vi "NI OCR-Start Training.vi"(8 "error in":errorcluster, 11 "Buffer Data In":T1={"VI Refnum"=refnum, "Src Image"=refnum, "Dst Image"=refnum, "Ctl Refnum []"=[], "Ctl Label"=[], "User Event"=refnum, "Event Registration Refnum"=refnum, "Timeout"=0, "IMAQ OCR Session"=refnum, "Objects"=[], "ROI Descriptor"={"Global Rectangle"=[], "Contours"=[]}, "Settings"={"Objects"=0, "Threshold"=128, "Reject Border"=FALSE, "Fill Holes"=FALSE, "Min Object Size"=FALSE, "Min Size"=3, "Max Object Size"=FALSE, "Max Size"=100, "Show Search Area"=FALSE, "Show Center"=TRUE, "Show Bounding Box"=TRUE}} {"Settings"."Objects" items=["Bright Objects", "Dark Objects"]; "Settings"."Threshold" min=1 max=999999999 step=1; "Settings"."Max Size" min=1 max=999999999 step=1; "Settings"."Min Size" min=1 max=999999999 step=1; "ROI Descriptor"."Contours"."Type" items=["No Selection", "Point", "Line", "Rectangle", "Oval", "Polygon", "Freehand Region", "Annulus", "Unused2", "Unused3", "Broken Line", "Freehand Line", "Rotated Rectangle"]; "Objects"."Aspect Ratio" format="%.2f"; "Objects"."Orientation" format="%.2f"; "Objects"."Area" format="%.2f"; "Objects"."Object Center"."Y" format="%.2f"; "Objects"."Object Center"."X" format="%.2f"}) -> (0 "error out":errorcluster, 3 "Buffer Data Out":T1={"VI Refnum"=refnum, "Src Image"=refnum, "Dst Image"=refnum, "Ctl Refnum []"=[], "Ctl Label"=[], "User Event"=refnum, "Event Registration Refnum"=refnum, "Timeout"=0, "IMAQ OCR Session"=refnum, "Objects"=[], "ROI Descriptor"={"Global Rectangle"=[], "Contours"=[]}, "Settings"={"Objects"=0, "Threshold"=128, "Reject Border"=FALSE, "Fill Holes"=FALSE, "Min Object Size"=FALSE, "Min Size"=3, "Max Object Size"=FALSE, "Max Size"=100, "Show Search Area"=FALSE, "Show Center"=TRUE, "Show Bounding Box"=TRUE}} {"Settings"."Objects" items=["Bright Objects", "Dark Objects"]; "Settings"."Threshold" min=1 max=999999999 step=1; "Settings"."Max Size" min=1 max=999999999 step=1; "Settings"."Min Size" min=1 max=999999999 step=1; "ROI Descriptor"."Contours"."Type" items=["No Selection", "Point", "Line", "Rectangle", "Oval", "Polygon", "Freehand Region", "Annulus", "Unused2", "Unused3", "Broken Line", "Freehand Line", "Rotated Rectangle"]; "Objects"."Aspect Ratio" format="%.2f"; "Objects"."Orientation" format="%.2f"; "Objects"."Area" format="%.2f"; "Objects"."Object Center"."Y" format="%.2f"; "Objects"."Object Center"."X" format="%.2f"})   [LabVIEW 2016]
uses:
  Data Def/NI OCR-Buffer Data.ctl
  <vilib>/vision/Image Controls.llb/IMAQ Image.ctl
  Data Def/NI OCR-User Event Data.ctl
  <vilib>/vision/OCR.llb/IMAQ OCR Session.ctl
  <vilib>/vision/NI_Vision_Development_Module.lvlib
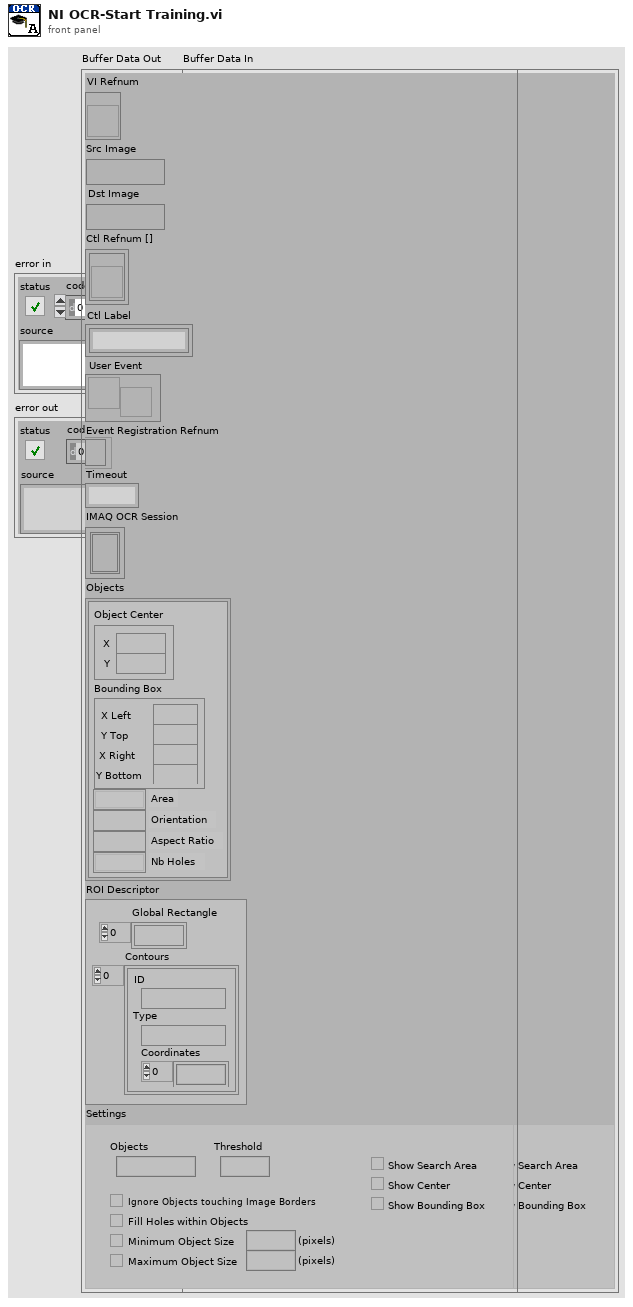
[diagram p1: front panel]
types:
  T1 = typedef "NI OCR-Buffer Data.ctl" = cluster{"VI Refnum":refnum<vi>, "Src Image":T2, "Dst Image":T2, "Ctl Refnum []":refnum<vi>[], "Ctl Label":string[], "User Event":refnum<user-event>, "Event Registration Refnum":refnum<event-registration>, "Timeout":i32, "IMAQ OCR Session":T3, "Objects":cluster{"Object Center":cluster{"X":sgl, "Y":sgl}, "Bounding Box":cluster{"X Left":i32, "Y Top":i32, "X Right":i32, "Y Bottom":i32}, "Area":sgl, "Orientation":sgl, "Aspect Ratio":sgl, "Nb Holes":i32}[], "ROI Descriptor":T4, "Settings":cluster{"Objects":u16, "Threshold":i32, "Reject Border":bool, "Fill Holes":bool, "Min Object Size":bool, "Min Size":i32, "Max Object Size":bool, "Max Size":i32, "Show Search Area":bool, "Show Center":bool, "Show Bounding Box":bool}}
  T2 = typedef "IMAQ Image.ctl" = refnum<image>
  T3 = typedef "IMAQ OCR Session.ctl" = refnum<k1>
  T4 = typedef "ROI Descriptor" = cluster{"Global Rectangle":i32[], "Contours":cluster{"ID":enum32{"External", "Internal"}, "Type":u32, "Coordinates":i32[]}[]}
  T5 = cluster{"Object Center":cluster{"X":sgl, "Y":sgl}, "Bounding Box":cluster{"X Left":i32, "Y Top":i32, "X Right":i32, "Y Bottom":i32}, "Area":sgl, "Orientation":sgl, "Aspect Ratio":sgl, "Nb Holes":i32}[]
  T6 = cluster{"X Left":i32, "Y Top":i32, "X Right":i32, "Y Bottom":i32}
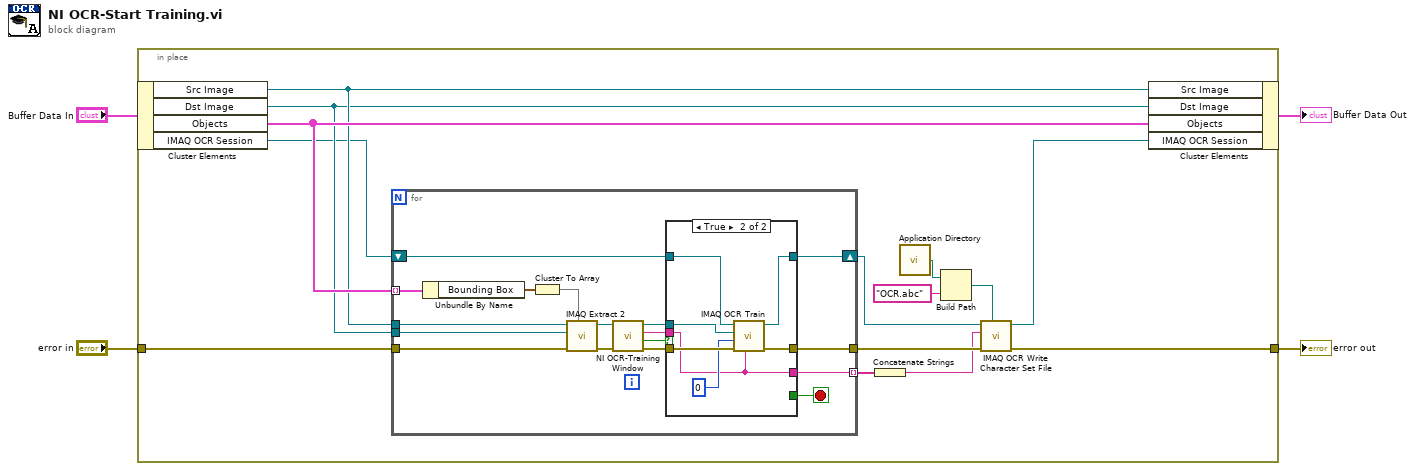
[diagram p0: block diagram]
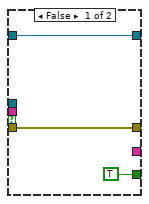
[diagram p2: hidden frame]
diagram:
  n1 = in-place {
    in-place-border: "error in" -> [w17]
    in-place-border: [w7] -> w1
    n2 = in-place-cluster #1("Buffer Data In") -> ("Src Image"=w16:T2, "Dst Image"=w15:T2, "Objects"=w18:T5, "IMAQ OCR Session"=w14:T3)
    n3 = for {
      tunnel: w18 -> [w35] mode=indexing
      tunnel: w17 -> [w34]
      tunnel: w16 -> [w32]
      tunnel: w15 -> [w33]
      shift-right: [w21] -> w10
      shift-left: w14 -> [w28]
      tunnel: [w20] -> w11
      tunnel: [w19] -> w6 mode=indexing
      stop <- w22 stop-if-true
      n4 = Unbundle By Name(w35) -> ("Bounding Box"=w31:T6)
      n5 = Cluster To Array(cluster=w31) -> (array=w30:i32[])
      n6 = call "IMAQ Extract 2"("Optional Rectangle"=w30, "error in (no error)"=w34, "Image Dst"=w33, "Image Src"=w32) -> ("error out"=w29:errorcluster, "Image Dst Out"=w27:T2)  [unwired: 6 in]
      n7 = call "NI OCR-Training Window.vi"("error in"=w29, "Image In"=w27) -> ("error out"=w25:errorcluster, "OK?"=w26:bool, "Character Out"=w23:string, "Image Out"=w24:T2)  [unwired: 6 in]
      n8 = case shown="True" w26 {
        tunnel: w28 -> [w37 w45]
        tunnel: w25 -> [w38 w43]
        tunnel: w24 -> [_ w44]
        tunnel: w23 -> [_ w39]
        tunnel: [w37 w42] -> w21
        tunnel: [w38 w41] -> w20
        tunnel: [TRUE _] -> w22
        tunnel: [_ w39] -> w19
        frame False {
        }
        frame True {
          n9 = call "IMAQ OCR Train"("Character Value"=w39, "error in (no error)"=w43, "Object Index"=0, "Image"=w44, "IMAQ OCR Session"=w45) -> ("error out"=w41:errorcluster, "IMAQ OCR Session (dup)"=w42:T3)  [unwired: 4 in, 1 out]
        }
      }
    }
    n10 = Concatenate Strings(w6) -> (w5:string)
    n11 = call <vilib>:"Application Directory.vi"() -> ("Application Directory"=w12:path)
    n12 = Build Path(base path=w12, name or relative path="OCR.abc") -> (appended path=w9:path)
    n13 = call "IMAQ OCR Write Character Set File"("File Path"=w9, "error in (no error)"=w11, "Character Set Description"=w5, "IMAQ OCR Session"=w10) -> ("error out"=w7:errorcluster, "IMAQ OCR Session (dup)"=w8:T3)  [unwired: 6 in]
    n14 = in-place-cluster #1("Src Image"=w16, "Dst Image"=w15, "Objects"=w18, "IMAQ OCR Session"=w8) -> (→"Buffer Data Out":T1)
  }
  "error out" <- w1
